vi "Create Plugin Configuration.vi"(6 "plugin timing":T2={"priority"=0, "decimation"=1, "offset"=0}, 8 "thread count":i32, 9 "settings":T1, 10 "group configs":T5(array[cluster]), 11 "plugin class":string) -> (3 "Plugin Configuration":T6={"name"="", "class"="", "cycle timing"={"priority"=0, "decimation"=1, "offset"=0}, "Transfer Groups"=[], "settings"=[], "thread count"=1} {"Transfer Groups"."Transfers"."channel configurations"."buffer offset" format="%d bytes"})   [LabVIEW 2017]
uses:
  Builds/Data Sharing Framework/Current/Data Sharing Framework Core/DSF Core.lvlibp/Configuration/Public/Controls/DSF Engine Plugin Configuration.ctl
  Builds/Data Sharing Framework/Current/Data Sharing Framework Core/DSF Core.lvlibp/Configuration/Public/Controls/DSF Timing Info.ctl
  Builds/Data Sharing Framework/Current/Data Sharing Framework Core/DSF Core.lvlibp/Configuration/Public/Controls/DSF Engine Transfer Group Configuration.ctl
  Builds/Data Sharing Framework/Current/Data Sharing Framework Core/DSF Core.lvlibp/Configuration/Public/Controls/DSF Direction.ctl
  Builds/Data Sharing Framework/Current/Data Sharing Framework Core/DSF Core.lvlibp/Configuration/Public/Controls/DSF Engine Transfer Configuration.ctl
  Builds/Data Sharing Framework/Current/Data Sharing Framework Core/DSF Core.lvlibp/Configuration/Public/Controls/DSF Byte Order.ctl
  Builds/Data Sharing Framework/Current/Data Sharing Framework Core/DSF Core.lvlibp/Configuration/Public/Controls/DSF Engine Channel Configuration.ctl
  Builds/Data Sharing Framework/Current/Data Sharing Framework Core/DSF Core.lvlibp/Configuration/Public/Controls/DSF Data Type.ctl
  Builds/Data Sharing Framework/Current/Data Sharing Framework Core/DSF Core.lvlibp/Configuration/Public/Controls/DSF Settings Info.ctl
  Builds/Data Sharing Framework/Current/Data Sharing Framework Core/DSF Core.lvlibp
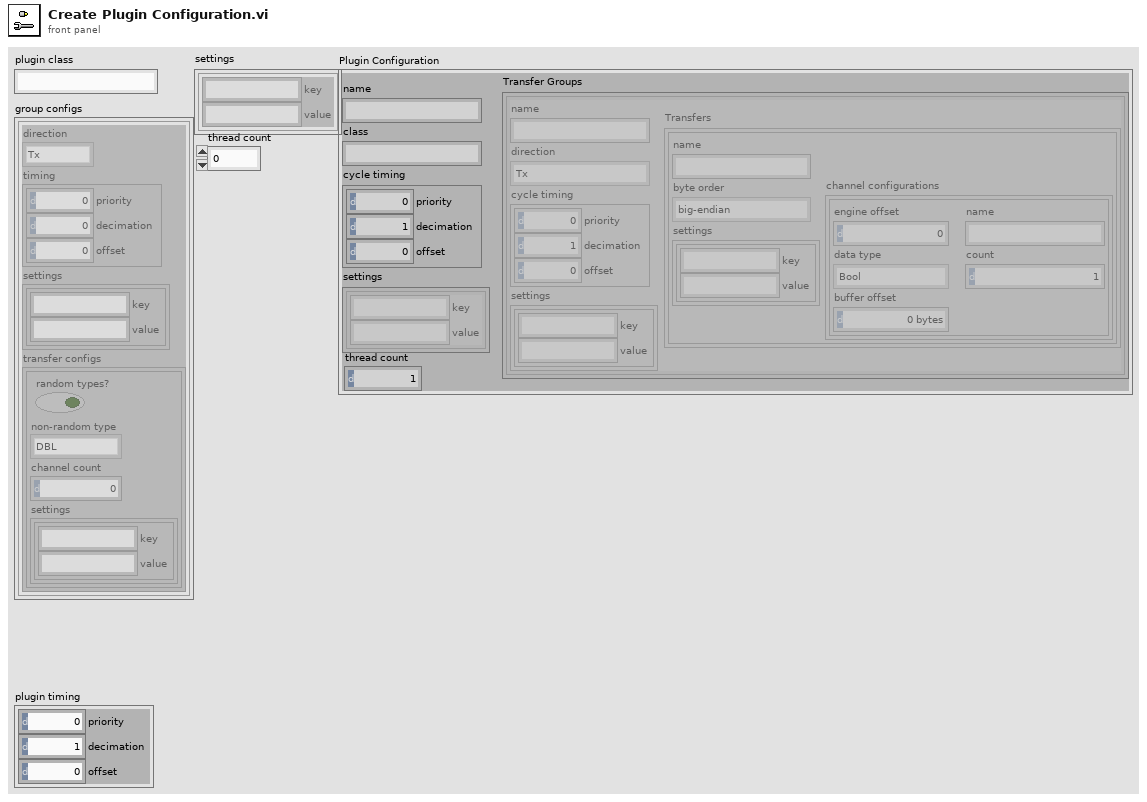
[diagram p1: front panel]
types:
  T1 = typedef "DSF Core.lvlibp/DSF Settings Info.ctl" = cluster{"key":string, "value":string}[]
  T2 = typedef "DSF Core.lvlibp/DSF Timing Info.ctl" = cluster{"priority":u64, "decimation":u64, "offset":u64}
  T3 = typedef "DSF Core.lvlibp/DSF Direction.ctl" = enum8{"Tx", "Rx"}
  T4 = typedef "DSF Core.lvlibp/DSF Data Type.ctl" = enum8{"Bool", "SGL", "DBL", "I8", "I16", "I32", "I64", "U8", "U16", "U32", "U64"}
  T5 = cluster{"direction":T3, "timing":T2, "settings":T1, "transfer configs":cluster{"random types?":bool, "non-random type":T4, "channel count":i32, "settings":T1}[]}[]
  T6 = typedef "DSF Core.lvlibp/DSF Engine Plugin Configuration.ctl" = cluster{"name":string, "class":string, "cycle timing":T2, "Transfer Groups":T7[], "settings":T1, "thread count":i32}
  T7 = typedef "DSF Core.lvlibp/DSF Engine Transfer Group Configuration.ctl" = cluster{"name":string, "direction":T3, "cycle timing":T2, "Transfers":T8[], "settings":T1}
  T8 = typedef "DSF Core.lvlibp/DSF Engine Transfer Configuration.ctl" = cluster{"name":string, "byte order":T9, "channel configurations":T10[], "settings":T1}
  T9 = typedef "DSF Core.lvlibp/DSF Byte Order.ctl" = enum8{"big-endian", "little-endian"}
  T10 = typedef "DSF Core.lvlibp/DSF Engine Channel Configuration.ctl" = cluster{"engine offset":u64, "name":string, "data type":T4, "count":u64, "buffer offset":u64}
  T11 = cluster{"random types?":bool, "non-random type":T4, "channel count":i32, "settings":T1}[]
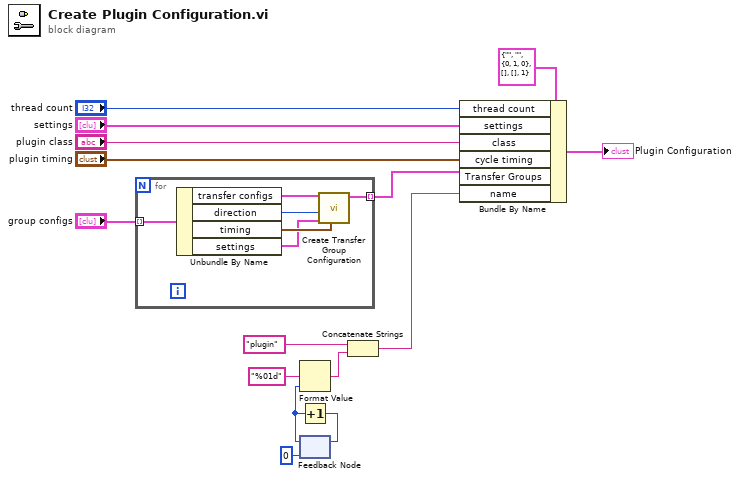
[diagram p0: block diagram]
diagram:
  n1 = for {
    tunnel: [w21] -> w4 mode=indexing
    tunnel: "group configs" -> [w20] mode=indexing
    n2 = Unbundle By Name(w20) -> ("transfer configs"=w16:T11, "direction"=w18:T3, "timing"=w19:T2, "settings"=w17:T1)
    n3 = call "Create Transfer Group Configuration.vi"("group timing (dec:1, off: 0)"=w19, "settings"=w17, "direction"=w18, "transfer configs"=w16) -> ("Transfer Group"=w21:T7)  [unwired: 7 in]
  }
  n4 = feedback #1(0) -> (w13:i32)
  n5 = Format Value(format string="%01d", value (0)=w13) -> (output string=w10:string)  [unwired: 1 in]
  n6 = Increment(x=w13) -> (x+1=w14:i32)
  n7 = feedback-in #1(w14) -> ()
  n8 = Concatenate Strings("plugin" ("name"), w10) -> (w7:string)
  n9 = Bundle By Name(cluster=T6 {"name"="", "class"="", "cycle timing"={"priority"=0, "decimation"=1, "offset"=0}, "Transfer Groups"=[], "settings"=[], "thread count"=1} ("Plugins 2"), "thread count"="thread count", "settings"="settings", "class"="plugin class", "cycle timing"="plugin timing", "Transfer Groups"=w4, "name"=w7) -> (→"Plugin Configuration":T6)
